vi "Task 1 calc.vi"() -> ()   [LabVIEW 2021]
panel:
  in  "=":bool
  out "Result":dbl
  in  "Num 2":dbl
  in  "Num 1":dbl
  in  "Enum":enum16{"Add", "Subtract", "Multiply", "Divide"}(ring)
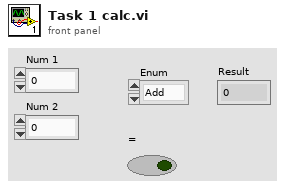
[diagram p1: front panel]
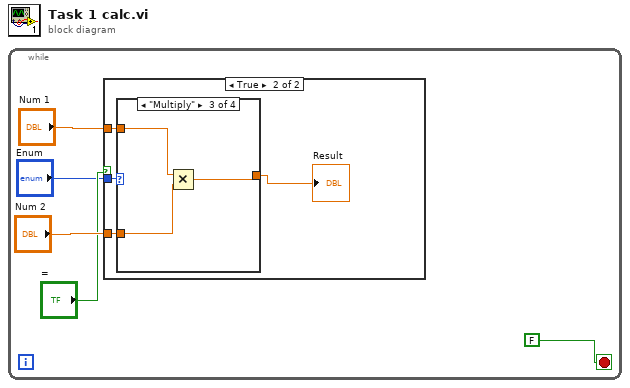
[diagram p0: block diagram]
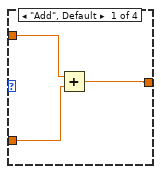
[diagram p3: hidden frame]
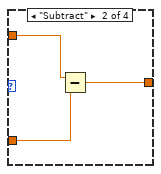
[diagram p4: hidden frame]
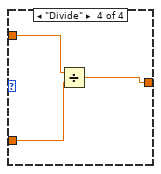
[diagram p5: hidden frame]
diagram:
  n1 = while {
    stop <- FALSE stop-if-true
    n2 = case shown="True" "=" {
      tunnel: "Num 1" -> [_ w9]
      tunnel: "Num 2" -> [_ w8]
      tunnel: "Enum" -> [_ w7]
      frame False {
      }
      frame True {
        n3 = case shown="\"Multiply\"" w7 {
          tunnel: w9 -> [w12 w15 w18 w21]
          tunnel: w8 -> [w11 w14 w17 w20]
          tunnel: [w10 w13 w16 w19] -> w6
          frame "Add", Default {
            n4 = Add(x=w12, y=w11) -> (x+y=w10:dbl)
          }
          frame "Subtract" {
            n5 = Subtract(x=w15, y=w14) -> (x-y=w13:dbl)
          }
          frame "Multiply" {
            n6 = Multiply(x=w18, y=w17) -> (x*y=w16:dbl)
          }
          frame "Divide" {
            n7 = Divide(x=w21, y=w20) -> (x/y=w19:dbl)
          }
        }
        "Result" <- w6
      }
    }
  }
